vi "Save to CSV.vi"(1 "Q":dbl[](array[numeric]), 2 "file name":string, 3 "I":dbl[](array[numeric])) -> ()   [LabVIEW 2024]
uses:
  <vilib>/Utility/file.llb/Write Delimited Spreadsheet (DBL).vi
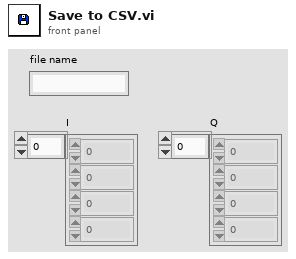
[diagram p1: front panel]
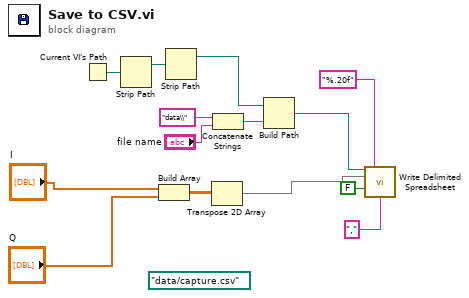
[diagram p0: block diagram]
diagram:
  (unwired) path "data/capture.csv" ("file path (dialog if empty)")
  n1 = Current VI's Path() -> (path=w9:path)
  n2 = Strip Path(path=w9) -> (stripped path=w6:path)  [unwired: 1 out]
  n3 = Build Array("I", "Q") -> (w8:dbl[][])
  n4 = Strip Path(path=w6) -> (stripped path=w5:path)  [unwired: 1 out]
  n5 = Transpose 2D Array(2D array=w8) -> (transposed array=w7:dbl[][])
  n6 = Concatenate Strings("data\\", "file name") -> (w1:string)
  n7 = Build Path(base path=w5, name or relative path=w1) -> (appended path=w10:path)
  n8 = call-poly <vilib>:"Write Delimited Spreadsheet.vi"("file path (dialog if empty)"=w10, "format (%.3f)"="%.20f", "2D data"=w7, "append to file? (new file:F)"=FALSE, "delimiter (\\t)"="," ("delimiter (\\t)")) -> ()  [unwired: 9 in, 2 out]
